vi "Z_CONT.vi"(8 "error in (no error)":errorcluster, 9 "element":T1 {"Avoid zero threshold (V)" format="%#_13g"}, 10 "ScanQ in":refnum<queue>, 11 "Queue in":refnum<queue>) -> (0 "error out":errorcluster, 2 "Z-Controller on/off status":bool, 3 "Queue out":refnum<queue>)   [LabVIEW 2025]
uses:
  <userlib>/Nanonis Prog Interface V5e/Nanonis Prog Interface.lvlib
  STM-Auto-Project/QMH CTLS/Scan_Params (QMH).ctl
  Downloads/OneDrive_2025-09-03/Instrument Controls/Temp Cntrl.ctl
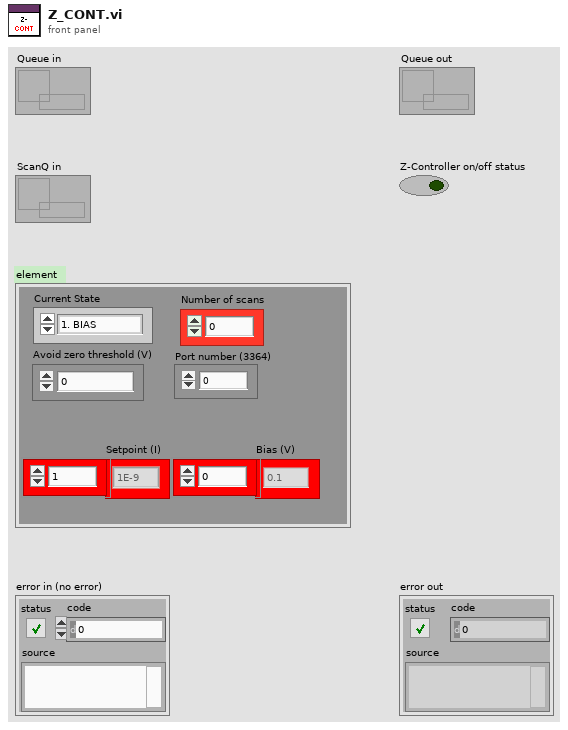
[diagram p1: front panel]
types:
  T1 = typedef "Scan_Params (QMH).ctl" = cluster{"Setpoint (I)":dbl[], "Bias (V)":dbl[], "Number of scans":u8, "Port number (3364)":u32, "Avoid zero threshold (V)":dbl, "Current State":enum16{"1. BIAS", "2. INIT_SCAN", "3. SCAN_IDLE", "4. INTER_SCAN", "5. NEW_COORDS_&_FRAME", "6. FINAL_SCAN", "7. POLL BIAS ", "8. Z-CONT.", "9. STOP"}}
  T2 = enum16{"1. BIAS", "2. INIT_SCAN", "3. SCAN_IDLE", "4. INTER_SCAN", "5. NEW_COORDS_&_FRAME", "6. FINAL_SCAN", "7. POLL BIAS ", "8. Z-CONT.", "9. STOP"}
  T3 = enum16{"1. INIT TEMP", "2. TC ON", "3. POLL_TEMPS", "4. TEMP_STAB", "5. TC IDLE", "6. APPLY NEXT TEMP", "7. TC OFF (Reset)"}
  T4 = typedef "Temp Cntrl.ctl" = cluster{"Range (0:Off)":u16, "Manual Output (0.00 %)":dbl, "Rate (D) (0.0 %)":dbl, "Reset (I) (20.0)":dbl, "Gain (P) (50.0)":dbl, "Power Up Enable (F: Disable)":bool, "Max User Current (2.000)":dbl, "Heater Resistance (1:25 Ohms)":u16, "Max Current (0:User Specified)":u16, "Heater Out Display (1:Current)":u16, "Mode (0:Off)":u16, "Input (0:None)":u16, "Target Temp (K)":dbl, "Serial Configuration":cluster{"Baud Rate":u32, "Parity":u16, "Data Bits":u16, "Stop Bits":u16, "Flow Control":u16}, "VISA resource name":refnum<visa-resource-name>, "Configure Control Parameters (0: Configure)":u16, "Enable Setpoint (F:Disable)":bool, "Input (0:A)":u16, "Data Source (0:Kelvin)":u16, "Output's Control Loop (1:1)":u16, "STND DEV Threshold ":dbl, "Mean Tolerance ":dbl, "Current State":enum16{"1. INIT TEMP", "2. TC ON", "3. POLL_TEMPS", "4. TEMP_STAB", "5. TC IDLE", "6. APPLY NEXT TEMP", "7. TC OFF (Reset)"}}
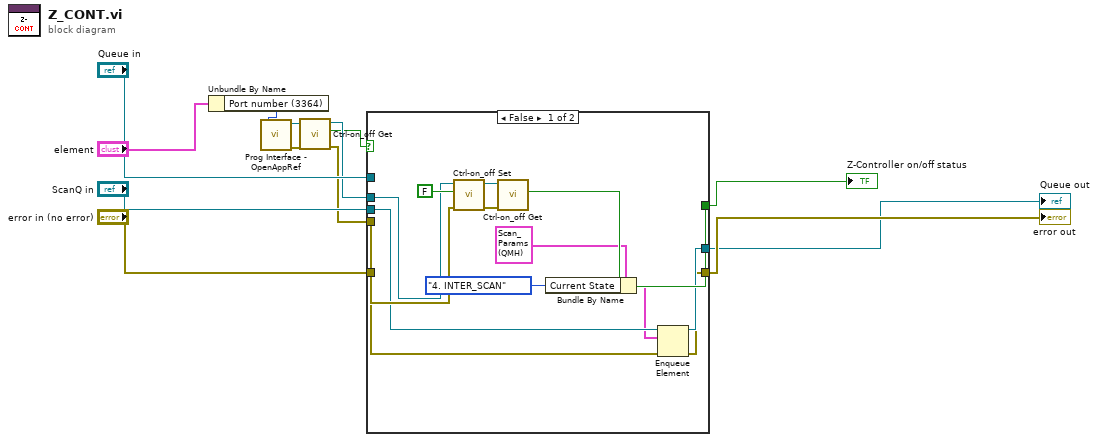
[diagram p0: block diagram]
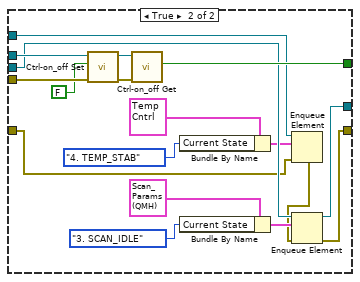
[diagram p2: hidden frame]
diagram:
  n1 = Unbundle By Name("element") -> ("Port number (3364)"=w13:u32)
  n2 = call <userlib>:"Prog Interface - OpenAppRef.vi"("Port number (3364)"=w13) -> ("Error out"=w10:errorcluster, "Application reference"=w11:refnum<vi>)  [unwired: 5 in]
  n3 = call <userlib>:"Ctrl-on_off Get.vi"("error in (no error)"=w10, "Application ref in"=w11) -> ("error out"=w3:errorcluster, "Z-Controller on/off status"=w1:bool, "Application ref out"=w2:refnum<vi>)  [unwired: 7 in]
  n4 = case shown="False" w1 {
    tunnel: w2 -> [w23 w44]
    tunnel: w3 -> [w22 w43]
    tunnel: [w21 w39] -> w4
    tunnel: "ScanQ in" -> [w20 w38]
    tunnel: [w16 w34] -> w6
    tunnel: [w15 w33] -> w7
    tunnel: "error in (no error)" -> [w14 w28]
    tunnel: "Queue in" -> [_ w32]
    frame False {
      n5 = call <userlib>:"Ctrl-on_off Set.vi"("error in (no error)"=w22, "Z Controller ON/OFF"=FALSE, "Application ref in"=w23) -> ("error out"=w25:errorcluster, "Application ref out"=w24:refnum<vi>)  [unwired: 7 in]
      n6 = call <userlib>:"Ctrl-on_off Get.vi"("error in (no error)"=w25, "Application ref in"=w24) -> ("Z-Controller on/off status"=w21:bool)  [unwired: 7 in, 2 out]
      n7 = Bundle By Name(cluster=T1 {"Setpoint (I)"=[], "Bias (V)"=[], "Number of scans"=1, "Port number (3364)"=3364, "Avoid zero threshold (V)"=0.004999999888241291, "Current State"=enum."1. BIAS"} ("element"), "Current State"=T2."4. INTER_SCAN") -> (w18:T1)
      n8 = Enqueue Element(queue=w20, element=w18, error in (no error)=w14) -> (queue out=w16:refnum<queue>, error out=w15:errorcluster)  [unwired: 1 in, 1 out]
    }
    frame True {
      n9 = call <userlib>:"Ctrl-on_off Set.vi"("error in (no error)"=w43, "Z Controller ON/OFF"=FALSE, "Application ref in"=w44) -> ("error out"=w41:errorcluster, "Application ref out"=w40:refnum<vi>)  [unwired: 7 in]
      n10 = call <userlib>:"Ctrl-on_off Get.vi"("error in (no error)"=w41, "Application ref in"=w40) -> ("Z-Controller on/off status"=w39:bool)  [unwired: 7 in, 2 out]
      n11 = Bundle By Name(cluster=T4 {"Range (0:Off)"=0, "Manual Output (0.00 %)"=0.0, "Rate (D) (0.0 %)"=0.0, "Reset (I) (20.0)"=20.0, "Gain (P) (50.0)"=50.0, "Power Up Enable (F: Disable)"=FALSE, "Max User Current (2.000)"=2.0, "Heater Resistance (1:25 Ohms)"=1, "Max Current (0:User Specified)"=0, "Heater Out Display (1:Current)"=1, "Mode (0:Off)"=1, "Input (0:None)"=4, "Target Temp (K)"=5.0, "Serial Configuration"={"Baud Rate"=57600, "Parity"=1, "Data Bits"=7, "Stop Bits"=10, "Flow Control"=0}, "VISA resource name"="", "Configure Control Parameters (0: Configure)"=0, "Enable Setpoint (F:Disable)"=FALSE, "Input (0:A)"=3, "Data Source (0:Kelvin)"=0, "Output's Control Loop (1:1)"=2, "STND DEV Threshold "=0.1, "Mean Tolerance "=0.02, "Current State"=enum."1. INIT TEMP"} ("element"), "Current State"=T3."4. TEMP_STAB") -> (w31:T4)
      n12 = Bundle By Name(cluster=T1 {"Setpoint (I)"=[], "Bias (V)"=[], "Number of scans"=1, "Port number (3364)"=3364, "Avoid zero threshold (V)"=0.004999999888241291, "Current State"=enum."1. BIAS"} ("element"), "Current State"=T2."3. SCAN_IDLE") -> (w36:T1)
      n13 = Enqueue Element(queue=w32, element=w31, error in (no error)=w28) -> (error out=w27:errorcluster)  [unwired: 1 in, 2 out]
      n14 = Enqueue Element(queue=w38, element=w36, error in (no error)=w27) -> (queue out=w34:refnum<queue>, error out=w33:errorcluster)  [unwired: 1 in, 1 out]
    }
  }
  "error out" <- w7
  "Queue out" <- w6
  "Z-Controller on/off status" <- w4
